vi "GFGstringGet.vi"(7 "GFG Refnum (use when calling from external project)":refnum<vi>, 11 "Variable Name in":string) -> (2 "Found/Replaced":bool, 3 "String":string)   [LabVIEW 2012, in "GFG library.lvlib"]
doc: "SciScan 1.2 160622"
uses:
  GFG library.lvlib
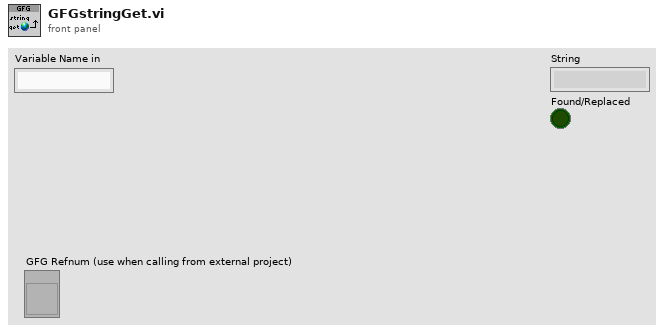
[diagram p1: front panel]
types:
  T1 = typedef "VariantType.lvlib/Type.ctl" = enum8{"Invalid Type", "Void", "I8", "I16", "I32", "I64", "U8", "U16", "U32", "U64", "Single Float", "Double Float", "Extended Float", "Single Complex", "Double Complex", "Extended Complex", "Enum U8", "Enum U16", "Enum U32", "Enum U64", "Single Float With Unit", "Double Float With Unit", "Extended Float With Unit", "Single Complex with Unit", "Double Complex with Unit", "Extended Complex with Unit", "Boolean", "String", "Path", "Picture", "Tag", "Array", "Cluster", "Variant", "LV Variant", "Waveform", "Timestamp", "Digital Waveform", "Digital Data", "ExpressData", "Refnum", "External Data", "VI", "Poly VI", "LabVIEW Class Instance", "Fixed Point"}
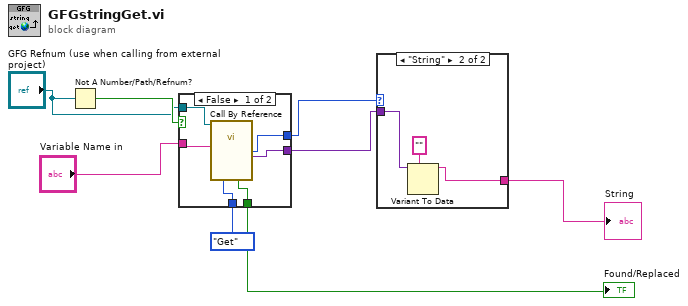
[diagram p0: block diagram]
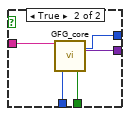
[diagram p2: hidden frame]
diagram:
  n1 = Not A Number/Path/Refnum?(number/path/refnum="GFG Refnum (use when calling from external project)") -> (NaN/Path/Refnum?=w6:bool)
  n2 = case shown="False" w6 {
    tunnel: enum16{"Init", "Set", "Get"}."Get" ("Action") -> [w11 w19]
    tunnel: "Variable Name in" -> [w12 w18]
    tunnel: [w13 w17] -> w2
    tunnel: [w14 w16] -> w3
    tunnel: "GFG Refnum (use when calling from external project)" -> [w10 _]
    tunnel: [w9 w15] -> w1
    frame False {
      n3 = call-by-ref "?"(reference=w10, "Variable Name in"=w12, "Action"=w11) -> ("Found/Replaced"=w9:bool, "Data Type Out"=w13:T1, "Variant Out"=w14:variant)  [unwired: 12 in, 6 out]
    }
    frame True {
      n4 = call "GFG_core.vi"("Variable Name in"=w18, "Action"=w19) -> ("Found/Replaced"=w15:bool, "Data Type Out"=w17:T1, "Variant Out"=w16:variant)  [unwired: 11 in, 4 out]
    }
  }
  "Found/Replaced" <- w1
  n5 = case shown="\"String\"" w2 {
    tunnel: w3 -> [_ w22]
    tunnel: [_ w20] -> w8
    frame Default {
    }
    frame "String" {
      n6 = Variant To Data(type="" ("Variable Name Out"), Variant=w22) -> (data=w20:string)  [unwired: 1 in, 1 out]
    }
  }
  "String" <- w8
